vi "GIP Example.vi"() -> ()   [LabVIEW 2021]
uses:
  controls/Signal Data.ctl
  controls/Frame Data.ctl
  <vilib>/xnet/xnet.llb/XNET Frame CAN.ctl
  <vilib>/xnet/xnet.llb/XNET Frame Type CAN.ctl
  support/CANbus/LunarSN.ctl
  controls/BCS Manager.ctl
panel:
  in  "Delay Time (s)":dbl=0.4 format="%#_13g"
  in  "Write Single Signal 2":T1[](array[typedef])
  in  "Lunar SN In":T2
  out "error out":errorcluster
  in  "Encode PN":bool
  in  "Encode SN":bool
  in  "Cyclic Period(ms)":i32
  in  "Write Frames":bool
  in  "Write Signals":bool
  in  "Write Single Frame":T3 {"Raw Frame"."payload" format="%x"; "Raw Frame"."timestamp" format="%<%.7X\n%x>T"; "Raw Frame"."type" items=["CAN Data"=0, "CAN Remote"=1, "CAN Bus Error"=2, "CAN 2.0 Data"=8, "CAN FD Data"=16, "CAN FD+BRS Data"=24, "J1939 Data"=192, "Delay"=224, "Log Trigger"=225, "Start Trigger"=226]; "Raw Frame"."identifier" format="%x"}
  in  "Write Single Signal":T1[](array[typedef])
  in  "Write Cyclic Frames":T3[](array[typedef]) {"Raw Frame"."payload" format="%x"; "Raw Frame"."timestamp" format="%<%.7X\n%x>T"; "Raw Frame"."type" items=["CAN Data"=0, "CAN Remote"=1, "CAN Bus Error"=2, "CAN 2.0 Data"=8, "CAN FD Data"=16, "CAN FD+BRS Data"=24, "J1939 Data"=192, "Delay"=224, "Log Trigger"=225, "Start Trigger"=226]; "Raw Frame"."identifier" format="%x"}
  in  "Write Cyclic Signals":T1[](array[typedef])
  out "Read Cyclic Frames":T3[](array[typedef]) {"Raw Frame"."payload" format="%x"; "Raw Frame"."timestamp" format="%<%.7X\n%x>T"; "Raw Frame"."type" items=["CAN Data"=0, "CAN Remote"=1, "CAN Bus Error"=2, "CAN 2.0 Data"=8, "CAN FD Data"=16, "CAN FD+BRS Data"=24, "J1939 Data"=192, "Delay"=224, "Log Trigger"=225, "Start Trigger"=226]; "Raw Frame"."identifier" format="%x"}
  out "Read Cyclic Signals":T1[](array[typedef])
  in  "stop":bool
  in  "DBC File":path=path "C:/Github/Testand_Template_x64/Config/CANbus/can_messages.dbc"
  in  "JSON signals file":path=path "C:/Github/Testand_Template_x64/Config/CANbus/GIP.json"
  # "-"
  # "-"
  # "-"
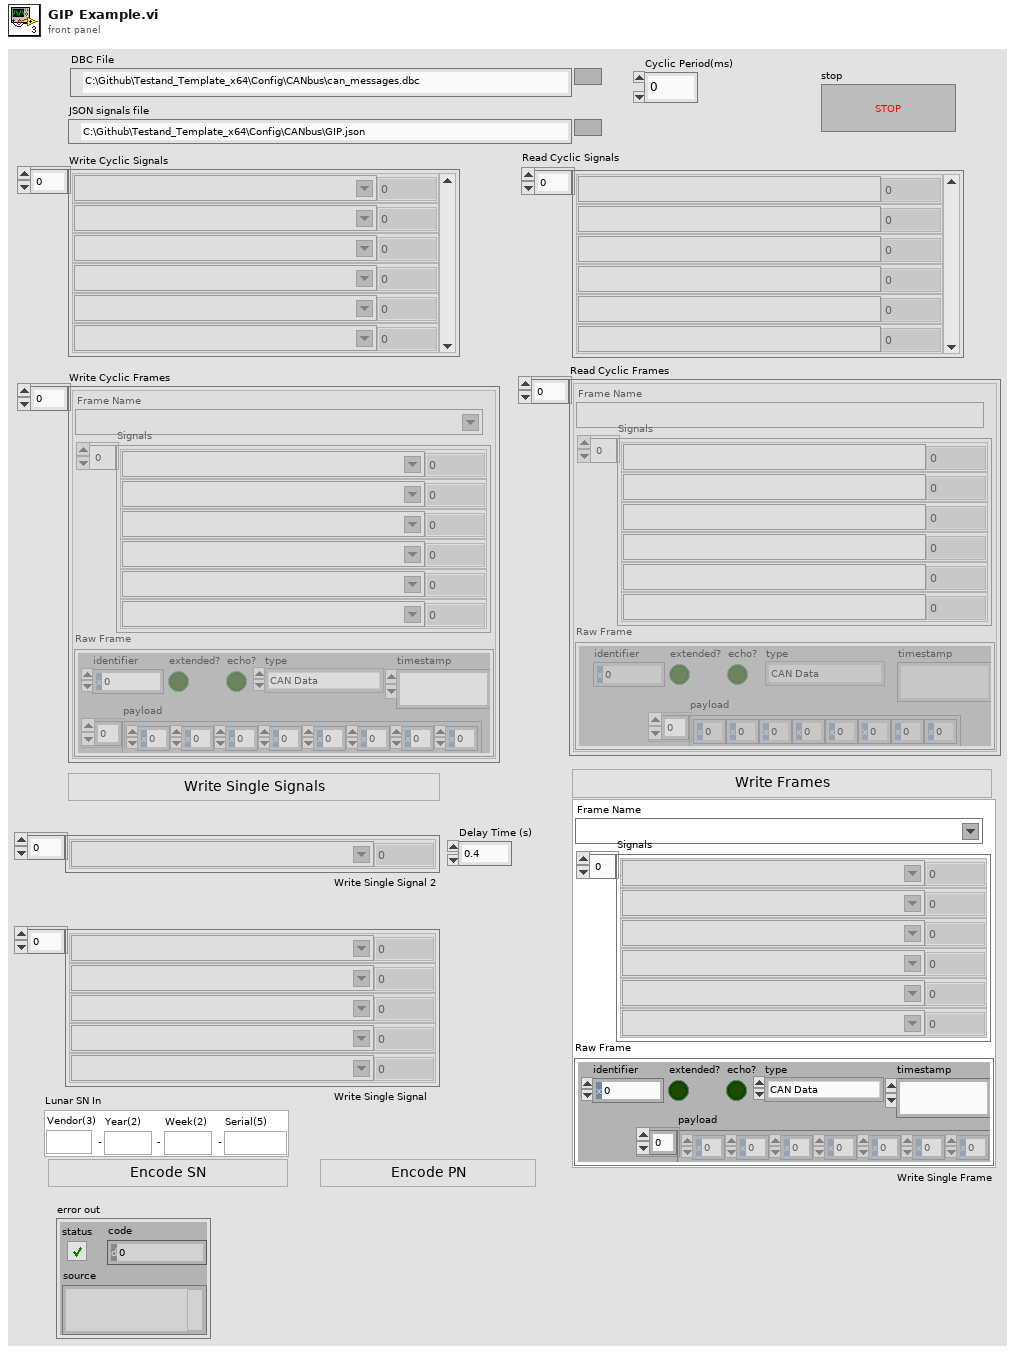
[diagram p1: front panel]
types:
  T1 = typedef "Signal Data.ctl" = cluster{"XNET Signal":refnum<k21>, "Data":dbl}
  T2 = typedef "LunarSN.ctl" = cluster{"Vendor(3)":string, "Year(2)":string, "Week(2)":string, "Serial(5)":string}
  T3 = typedef "Frame Data.ctl" = cluster{"Raw Frame":T4, "Frame Name":refnum<k21>, "Signals":T1[]}
  T4 = typedef "XNET Frame CAN.ctl" = cluster{"timestamp":timestamp, "payload":u8[], "identifier":u32, "type":T5, "extended?":bool, "echo?":bool}
  T5 = typedef "XNET Frame Type CAN.ctl" = u8
  T6 = typedef "BCS Manager.ctl" = enum16{"Init", "Start Signal Session", "Start Frame Session", "Write Sigs Session", "Write Frames Session", "Write Sigs Single", "Write Frames Single", "Read Sigs Session", "Read Frames Session", "Read Sigs Single", "Read Frames Single", "Write Raw Frame Session", "Write Raw Frame Single", "FrameRef to Sigs", "FrameID to FrameRef", "Close"}
  T7 = typedef "JSON sigs.ctl" = cluster{"Read Signals Cyclic":refnum<k21>[], "Write Signals Cyclic":refnum<k21>[], "Write Frames Cyclic":refnum<k21>[], "Read Frames Cyclic":refnum<k21>[]}
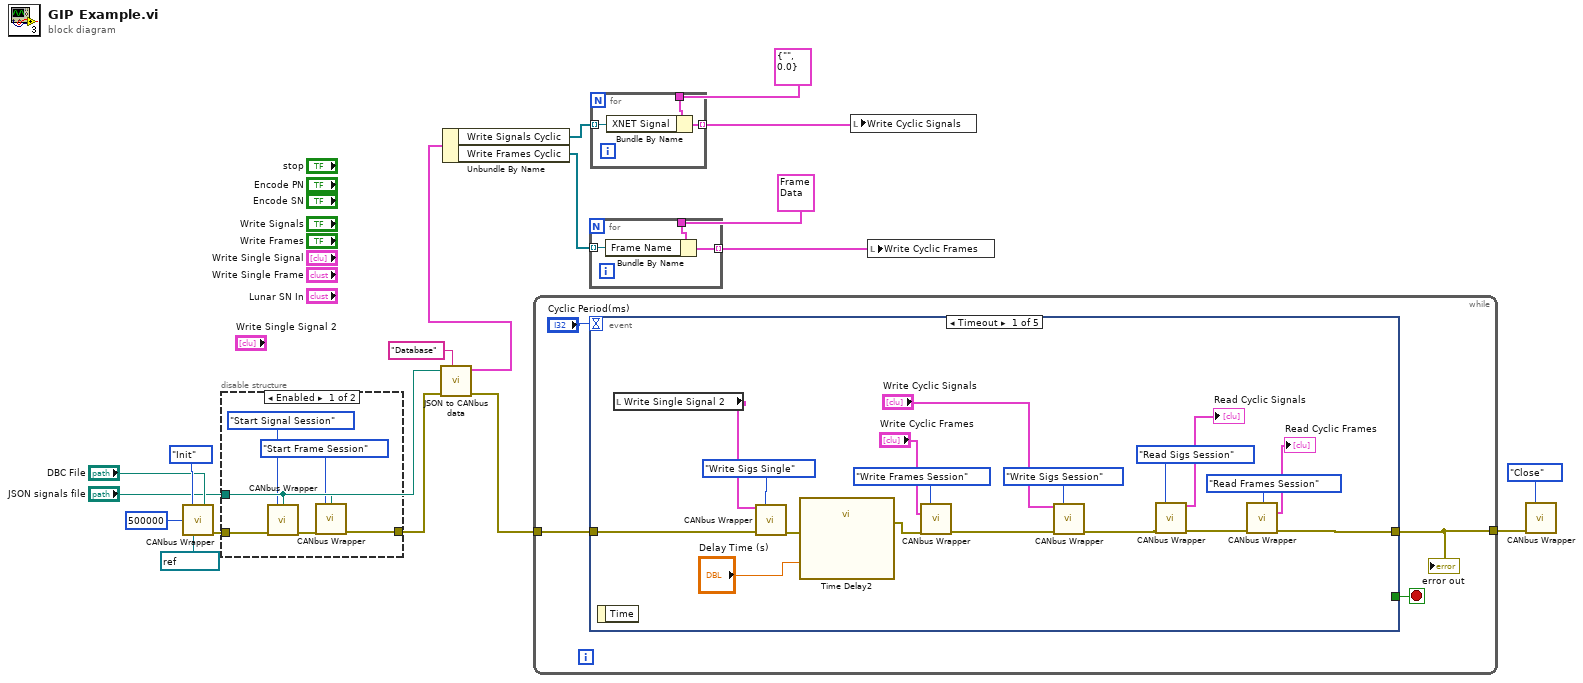
[diagram p0: block diagram]
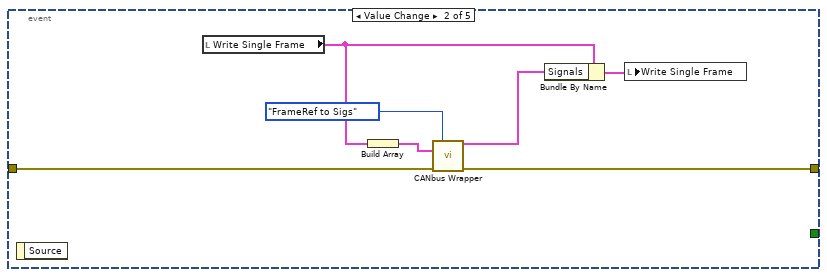
[diagram p3: hidden frame]
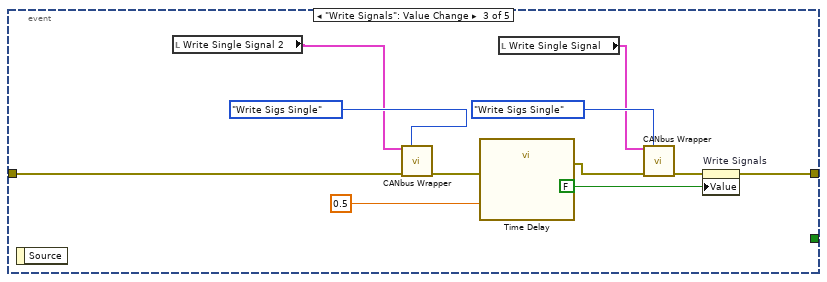
[diagram p4: hidden frame]
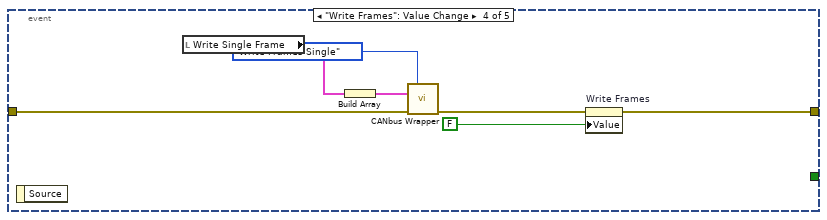
[diagram p5: hidden frame]
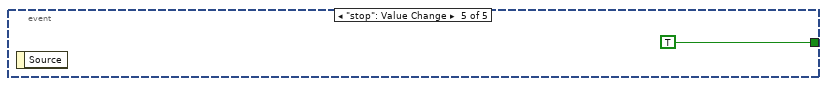
[diagram p6: hidden frame]
diagram:
  n1 = call "CANbus Wrapper.vi"("Method"=BCS_Manager."Init" ("Action"), "DBC File"="DBC File", "Baud Rate"=u64 500000, "interface"=refnum<k21> "CAN1") -> ("error out"=w17:errorcluster)  [unwired: 9 in, 2 out]
  n2 = disable-structure shown="Enabled" {
    disable-tunnel: w17 -> [w23 w25]
    disable-tunnel: "JSON signals file" -> [w20 _]
    disable-tunnel: [w19 w25] -> w1
    frame Enabled {
      n3 = call "CANbus Wrapper.vi"("Method"=BCS_Manager."Start Signal Session" ("Action"), "JSON signals file"=w20, "error in (no error)"=w23) -> ("error out"=w22:errorcluster)  [unwired: 10 in, 2 out]
      n4 = call "CANbus Wrapper.vi"("Method"=BCS_Manager."Start Frame Session", "JSON signals file"=w20, "error in (no error)"=w22) -> ("error out"=w19:errorcluster)  [unwired: 10 in, 2 out]
    }
    frame Disabled {
    }
  }
  n5 = call "JSON to CANbus data.vi"("Database Alias"="Database" ("database alias"), "error in"=w1, "JSON file"="JSON signals file") -> ("error out"=w9:errorcluster, "Signal Sessions"=w5:T7)  [unwired: 7 in]
  n6 = Unbundle By Name(w5) -> ("Write Signals Cyclic"=w4:refnum<k21>[], "Write Frames Cyclic"=w14:refnum<k21>[])
  n7 = while {
    tunnel: w9 -> [w29]
    tunnel: [w28] -> w7
    stop <- w26 stop-if-true
    n8 = event shown="[0] Timeout" {
      selector: _ -> [_ _ _ _ _]
      dyn-events: _ -> [_ _ _ _ _]
      timeout: "Cyclic Period(ms)" -> [_ _ _ _ _]
      tunnel: w29 -> [w34 w54 w60 w69 _]
      tunnel: [w44 w48 w62 w67 _] -> w28
      tunnel: [_ _ _ _ TRUE] -> w26
      event Timeout {
        n9 = event-data() -> ()  [unwired: 1 in, 1 out]
        n10 = local read "Write Single Signal 2"() -> (w35:T1[])
        n11 = call "CANbus Wrapper.vi"("Signals IN"=w35, "Method"=BCS_Manager."Write Sigs Single", "error in (no error)"=w34) -> ("error out"=w33:errorcluster)  [unwired: 10 in, 2 out]
        n12 = call "Time Delay2"("error in (no error)"=w33, "Delay Time (s)"="Delay Time (s)") -> ("error out"=w32:errorcluster)  [unwired: 9 in]
        n13 = call "CANbus Wrapper.vi"("Method"=BCS_Manager."Write Frames Session", "Frames IN"="Write Cyclic Frames", "error in (no error)"=w32) -> ("error out"=w37:errorcluster)  [unwired: 10 in, 2 out]
        n14 = call "CANbus Wrapper.vi"("Signals IN"="Write Cyclic Signals", "Method"=BCS_Manager."Write Sigs Session", "error in (no error)"=w37) -> ("error out"=w41:errorcluster)  [unwired: 10 in, 2 out]
        n15 = call "CANbus Wrapper.vi"("Method"=BCS_Manager."Read Sigs Session", "error in (no error)"=w41) -> ("Signals OUT"=→"Read Cyclic Signals":T1[], "error out"=w45:errorcluster)  [unwired: 11 in, 1 out]
        n16 = call "CANbus Wrapper.vi"("Method"=BCS_Manager."Read Frames Session", "error in (no error)"=w45) -> ("Frames OUT"=→"Read Cyclic Frames":T3[], "error out"=w44:errorcluster)  [unwired: 11 in, 1 out]
      }
      event Value Change {
        n17 = event-data() -> ()  [unwired: 1 in, 1 out]
        n18 = local read "Write Single Frame"() -> (w51:T3)
        n19 = Build Array(w51) -> (w52:T3[])
        n20 = call "CANbus Wrapper.vi"("Method"=BCS_Manager."FrameRef to Sigs", "Frames IN"=w52, "error in (no error)"=w54) -> ("Signals OUT"=w50:T1[], "error out"=w48:errorcluster)  [unwired: 10 in, 1 out]
        n21 = Bundle By Name(cluster=w51, "Signals"=w50) -> (w49:T3)
        n22 = local write "Write Single Frame"(w49) -> ()
      }
      event "Write Signals": Value Change {
        n23 = event-data() -> ()  [unwired: 1 in, 1 out]
        n24 = local read "Write Single Signal 2"() -> (w58:T1[])
        n25 = call "CANbus Wrapper.vi"("Signals IN"=w58, "Method"=BCS_Manager."Write Sigs Single", "error in (no error)"=w60) -> ("error out"=w57:errorcluster)  [unwired: 10 in, 2 out]
        n26 = call "Time Delay"("error in (no error)"=w57, "Delay Time (s)"=0.5) -> ("error out"=w56:errorcluster)  [unwired: 9 in]
        n27 = local read "Write Single Signal"() -> (w64:T1[])
        n28 = call "CANbus Wrapper.vi"("Signals IN"=w64, "Method"=BCS_Manager."Write Sigs Single", "error in (no error)"=w56) -> ("error out"=w63:errorcluster)  [unwired: 10 in, 2 out]
        n29 = property on="Write Signals" class="Bool (strict)"(error in=w63, "Value"=FALSE ("Send Signals")) -> (error out=w62:errorcluster)  [unwired: 1 in, 1 out]
      }
      event "Write Frames": Value Change {
        n30 = event-data() -> ()  [unwired: 1 in, 1 out]
        n31 = local read "Write Single Frame"() -> (w71:T3)
        n32 = Build Array(w71) -> (w70:T3[])
        n33 = call "CANbus Wrapper.vi"("Method"=BCS_Manager."Write Frames Single", "Frames IN"=w70, "error in (no error)"=w69) -> ("error out"=w68:errorcluster)  [unwired: 10 in, 2 out]
        n34 = property on="Write Frames" class="Bool (strict)"(error in=w68, "Value"=FALSE ("Write Frames")) -> (error out=w67:errorcluster)  [unwired: 1 in, 1 out]
      }
      event "stop": Value Change {
        n35 = event-data() -> ()  [unwired: 1 in, 1 out]
      }
    }
    "error out" <- w28
  }
  n36 = for {
    tunnel: w14 -> [w75] mode=indexing
    tunnel: T3 {"Raw Frame"={"timestamp"=timestamp(0 s since 1904-01-01), "payload"=[], "identifier"=0, "type"=0, "extended?"=FALSE, "echo?"=FALSE}, "Frame Name"="", "Signals"=[]} ("Frames IN") -> [w76]
    tunnel: [w74] -> w10 mode=indexing
    n37 = Bundle By Name(cluster=w76, "Frame Name"=w75) -> (w74:T3)
  }
  n38 = for {
    tunnel: w4 -> [w78] mode=indexing
    tunnel: T1 {"XNET Signal"="", "Data"=0.0} ("Signals IN") -> [w79]
    tunnel: [w77] -> w12 mode=indexing
    n39 = Bundle By Name(cluster=w79, "XNET Signal"=w78) -> (w77:T1)
  }
  n40 = local write "Write Cyclic Signals"(w12) -> ()
  n41 = local write "Write Cyclic Frames"(w10) -> ()
  n42 = call "CANbus Wrapper.vi"("Method"=BCS_Manager."Close", "error in (no error)"=w7) -> ()  [unwired: 11 in, 3 out]
